vi "Periodic Tasks.vi"(8 "error in":errorcluster) -> ()   [LabVIEW 2020]
doc: "This VI runs in parallel to other tasks. It can contain as many user-defined periodic loops as you need. These can carry out PID or other sorts of timed response."
uses:
  <vilib>/Rock Robotics/WPI/Utilities/WPI_GetSetVariantRefNum.vi
  Global Shooter Speed.vi
  <vilib>/Rock Robotics/WPI/ThirdParty/Phoenix-LabVIEW/CANCoder/Get/CTRE_Phoenix_CANcoder_GetSensorData.vi
  Auto Variables.vi
  <vilib>/Rock Robotics/Network Tables/NT Write Number.vi
panel:
  out "Gyro Angle":dbl
  # "Click here to set min"
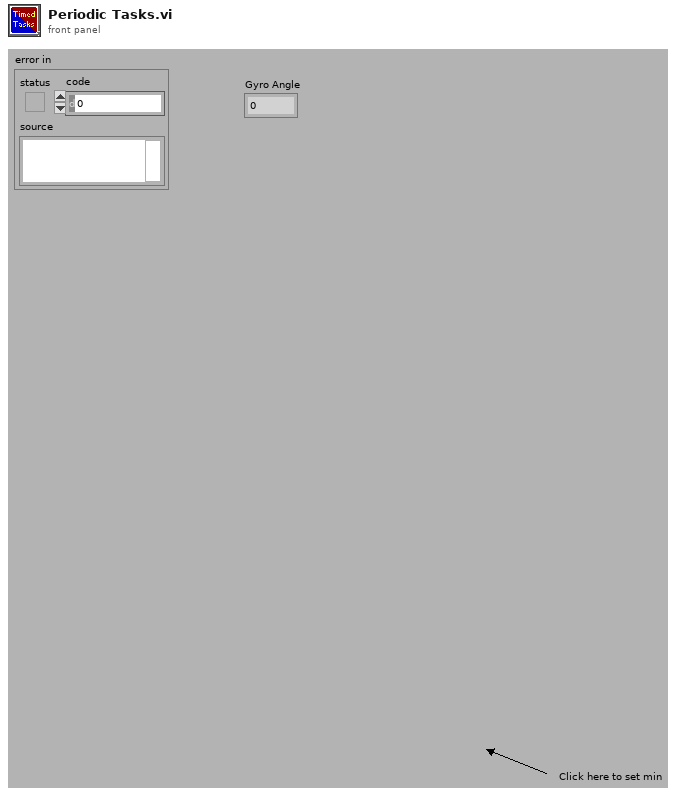
[diagram p1: front panel]
types:
  T1 = typedef "WPI_JoystickDevRef.ctl" = cluster{"Device":T2}
  T2 = typedef "WPI_JoystickDeviceEnum.ctl" = enum16{"USB 0", "USB 1", "USB 2", "USB 3", "USB 4", "USB 5"}
  T3 = typedef "WPI_RobotDriveDevRef.ctl" = cluster{"DevStatus":errorcluster, "Motors[]":T4[], "Square Inputs":bool, "Max Output":dbl}
  T4 = typedef "WPI_MotorControlDeviceRef.ctl" = cluster{"DeviceStatus":errorcluster, "Type":T5, "PWM":cluster{"PWM Channel":T6, "DeadBand":T7}, "CAN":cluster{"Device Number":u8, "SetOutput VI Ref":variant, "GetOutput VI Ref":variant, "Enable VI Ref":variant, "Disable VI Ref":variant, "Data":variant}, "Invert":bool, "DIO PWM":cluster{"PWM \"Enable\" Channel":T6, "DIOChannel":T8, "PWM Rate":dbl}}
  T5 = typedef "WPI_MotorControlType.ctl" = enum16{"PWM", "CAN", "DIO PWM"}
  T6 = typedef "FPGA_DIOPWMChannel.ctl" = enum8{"PWM 0", "PWM 1", "PWM 2", "PWM 3", "PWM 4", "PWM 5", "PWM 6", "PWM 7", "PWM 8", "PWM 9", "PWM MXP 0", "PWM MXP 1", "PWM MXP 2", "PWM MXP 3", "PWM MXP 4", "PWM MXP 5", "PWM MXP 6", "PWM MXP 7", "PWM MXP 8", "PWM MXP 9", "Invalid"}
  T7 = typedef "WPI_PWMDeadband.ctl" = cluster{"Name":string, "maxPositivePwm":i32, "minPositivePwm":i32, "centerPwm":i32, "maxNegativePwm":i32, "minNegativePwm":i32, "angularRange":u16}
  T8 = typedef "FPGA_DIOChannel.ctl" = enum8{"DIO 0", "DIO 1", "DIO 2", "DIO 3", "DIO 4", "DIO 5", "DIO 6", "DIO 7", "DIO 8", "DIO 9", "DIO MXP 0", "DIO MXP 1", "DIO MXP 2", "DIO MXP 3", "DIO MXP 4", "DIO MXP 5", "DIO MXP 6", "DIO MXP 7", "DIO MXP 8", "DIO MXP 9", "DIO MXP 10", "DIO MXP 11", "DIO MXP 12", "DIO MXP 13", "DIO MXP 14", "DIO MXP 15", "SPI Port CS1", "SPI Port CS2", "SPI Port CS3", "SPI Port MISO", "SPI Port MOSI", "Invalid"}
  T9 = typedef "CTRE_Phoenix_CANcoder_DeviceRef.ctl" = cluster{"DeviceStatus":errorcluster, "Device Number":u8, "Handle":u64, "UsageFrame":u32, "Library Path":path}
  T10 = cluster{"MotorControlDevRef":T4, "MotorControlDevRef":T4, "MotorControlDevRef":T4}
  T11 = cluster{"JoystickDevRef":T1, "JoystickDevRef":T1, "RobotDriveDevRef":T3}
  T12 = typedef "WPI_GyroDevRef.ctl" = cluster{"DevStatus":errorcluster, "Analog Channel":T13, "Gain (VoltsPerDegree/Second)":dbl, "Gyro Type":enum16{"Analog", "XRS450"}, "Handle":i32, "SPI Bus":T14, "Device Found":bool, "Sample Rate":dbl, "Calibrate On Open":bool, "Offset":dbl}
  T13 = typedef "FPGA_AIChannel.ctl" = enum8{"AI 0", "AI 1", "AI 2", "AI 3", "AI MXP 0", "AI MXP 1", "AI MXP 2", "AI MXP 3", "Invalid"}
  T14 = typedef "spi_bus.ctl" = enum16{"SPI On-Board, CS0", "SPI On-Board, CS1", "SPI On-Board, CS2", "SPI On-Board, CS3", "SPI MXP", "Invalid"}
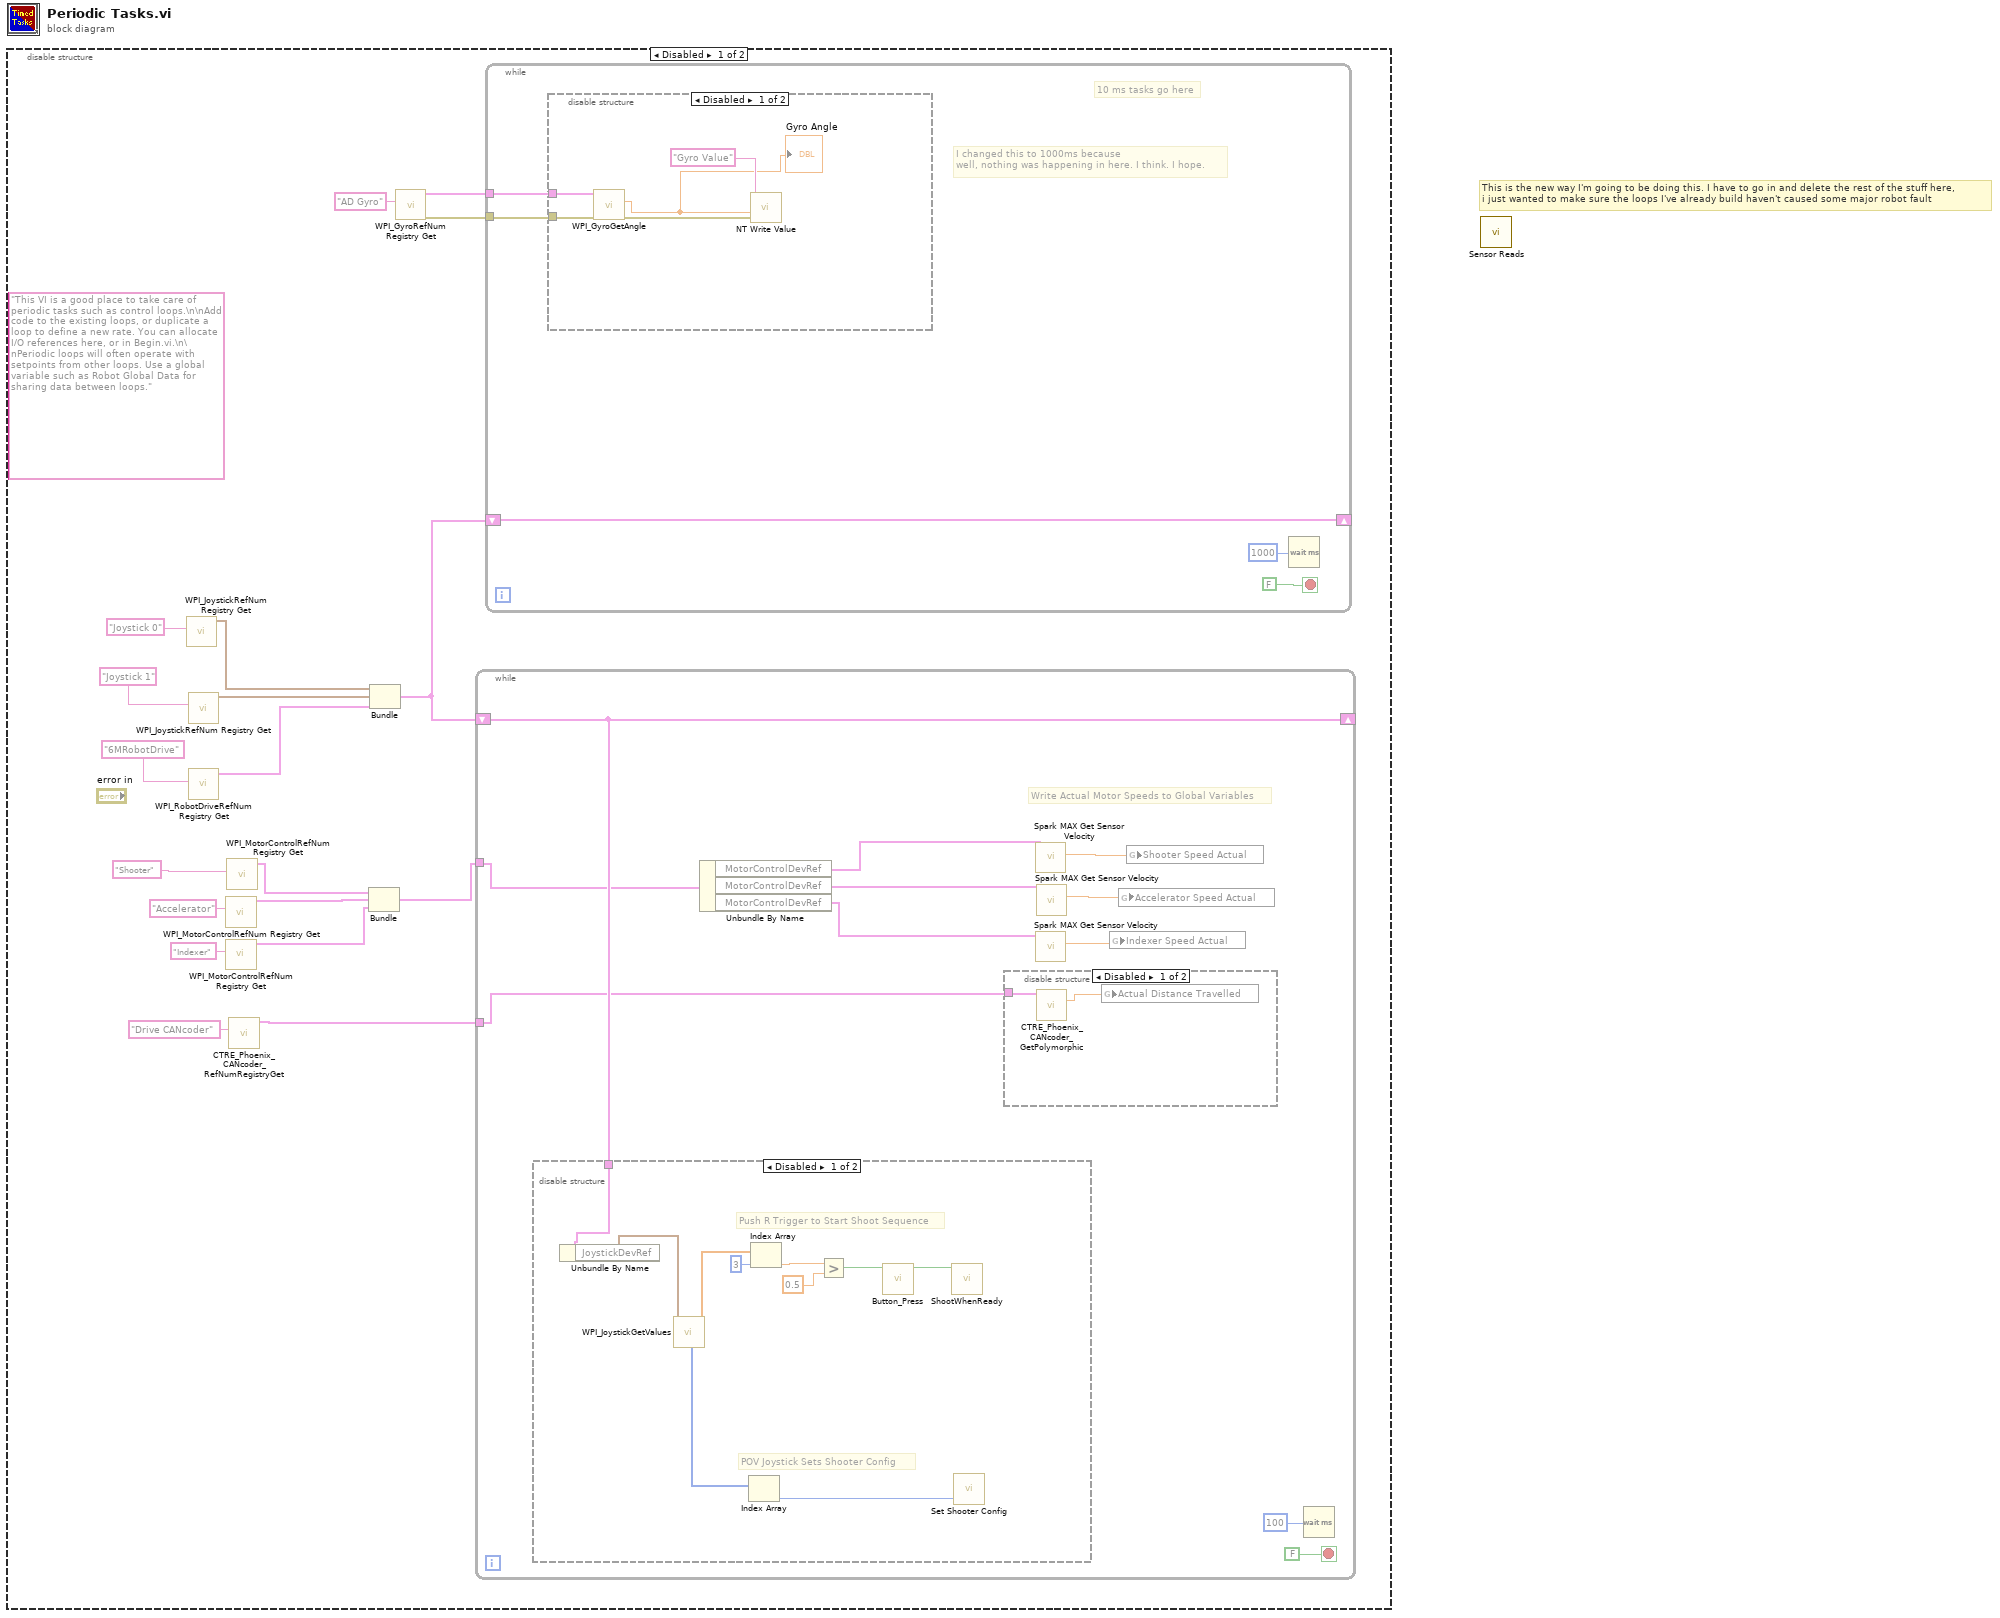
[diagram p0: block diagram]
diagram:
  # "This is the new way I'm going to be doing this. I have to go in and delete the rest of the stuff here,\ni just wanted to make sure the loops I've already build haven't caused some major robot fault"
  n1 = disable-structure shown="Disabled" {
    frame Disabled {
      (unwired) "This VI is a good place to take care of periodic tasks such as control loops.\n\nAdd code to the existing loops, or duplicate a loop to define a new rate. You can allocate I/O references here, or in Begin.vi.\n\nPeriodic loops will often operate with setpoints from other loops. Use a global variable such as Robot Global Data for sharing data between loops."
      n2 = call <vilib>:"WPI_JoystickRefNum Registry Get.vi"("refnum name"="Joystick 0") -> ("JoystickDevRef"=w13:T1)  [unwired: 9 in, 1 out]
      n3 = call <vilib>:"WPI_JoystickRefNum Registry Get.vi"("refnum name"="Joystick 1") -> ("JoystickDevRef"=w17:T1)  [unwired: 1 in, 9 out]
      n4 = call <vilib>:"WPI_RobotDriveRefNum Registry Get.vi"("refnum name"="6MRobotDrive") -> ("RobotDriveDevRef"=w16:T3)  [unwired: 1 in, 9 out]
      n5 = call <vilib>:"WPI_MotorControlRefNum Registry Get.vi"("refnum name"="Accelerator") -> ("MotorControlDevRef"=w6:T4)  [unwired: 9 in, 1 out]
      n6 = call <vilib>:"WPI_MotorControlRefNum Registry Get.vi"("refnum name"="Indexer") -> ("MotorControlDevRef"=w5:T4)  [unwired: 9 in, 1 out]
      n7 = call <vilib>:"WPI_MotorControlRefNum Registry Get.vi"("refnum name"="Shooter") -> ("MotorControlDevRef"=w7:T4)  [unwired: 9 in, 1 out]
      n8 = call <vilib>:"CTRE_Phoenix_CANcoder_RefNumRegistryGet.vi"("refnum name"="Drive CANcoder") -> ("CTRE_CANcoder_DeviceRef"=w8:T9)  [unwired: 9 in, 1 out]
      n9 = Bundle("MotorControlDevRef"=w7, "MotorControlDevRef"=w6, "MotorControlDevRef"=w5) -> (w4:T10)  [unwired: 1 in]
      n10 = Bundle("JoystickDevRef"=w13, "JoystickDevRef"=w17, "RobotDriveDevRef"=w16) -> (w15:T11)  [unwired: 1 out]
      n11 = call <vilib>:"WPI_GyroRefNum Registry Get.vi"("refnum name"="AD Gyro") -> ("error out"=w1:errorcluster, "GyroDevRef"=w2:T12)  [unwired: 9 in]
      n12 = while {
        shift-right: [w28] -> _
        shift-left: w15 -> [w28]
        tunnel: w4 -> [w23]
        tunnel: w8 -> [w24]
        stop <- FALSE stop-if-true
        # "Write Actual Motor Speeds to Global Variables"
        n13 = disable-structure shown="Disabled" {
          disable-tunnel: w28 -> [w40 _]
          frame Disabled {
            # "Push R Trigger to Start Shoot Sequence"
            # "POV Joystick Sets Shooter Config"
            n14 = Unbundle By Name(w40) -> ("JoystickDevRef"=w39:T1)
            n15 = call <vilib>:"WPI_JoystickGetValues.vi"("JoystickDevRef"=w39) -> ("Axes"=w36:dbl[], "POVs"=w38:i16[])  [unwired: 6 in, 3 out]
            n16 = Index Array(array=w38) -> (element=w37:i16)  [unwired: 1 in]
            n17 = Index Array(array=w36, index=3) -> (element=w34:dbl)
            n18 = Greater?(x=w34, y=0.5) -> (0:w32:bool)
            n19 = call "Button_Press.vi"("Button In"=w32) -> ("Button Pressed?"=w31:bool)  [unwired: 10 in]
            n20 = call "ShootWhenReady.vi"("Start Shooting"=w31) -> ()  [unwired: 11 in]
            n21 = call "Set Shooter Config.vi"("POV Joystick Input"=w37) -> ()  [unwired: 3 in]
          }
          frame Enabled {
          }
        }
        n22 = Unbundle By Name(w23) -> ("MotorControlDevRef"=w22:T4, "MotorControlDevRef"=w21:T4, "MotorControlDevRef"=w20:T4)
        n23 = disable-structure shown="Disabled" {
          disable-tunnel: w24 -> [w42 _]
          frame Disabled {
            n24 = call-poly <vilib>:"CTRE_Phoenix_CANcoder_GetPolymorphic.vi"("CTRE_CANcoder_DeviceRef"=w42) -> ("Position"=w41:dbl)  [unwired: 10 in, 4 out]
            n25 = global write "Auto Variables.vi" "Actual Distance Travelled"(w41) -> ()
          }
          frame Enabled {
          }
        }
        n26 = call <vilib>:"Spark MAX Get Sensor Velocity.vi"("MotorControlDevRef in"=w22) -> ("Sensor Velocity"=w27:dbl)  [unwired: 7 in, 3 out]
        n27 = call <vilib>:"Spark MAX Get Sensor Velocity.vi"("MotorControlDevRef in"=w20) -> ("Sensor Velocity"=w25:dbl)  [unwired: 7 in, 3 out]
        n28 = call <vilib>:"Spark MAX Get Sensor Velocity.vi"("MotorControlDevRef in"=w21) -> ("Sensor Velocity"=w26:dbl)  [unwired: 7 in, 3 out]
        n29 = global write "Global Shooter Speed.vi" "Indexer Speed Actual"(w25) -> ()
        n30 = global write "Global Shooter Speed.vi" "Accelerator Speed Actual"(w26) -> ()
        n31 = global write "Global Shooter Speed.vi" "Shooter Speed Actual"(w27) -> ()
        n32 = Wait (ms)(milliseconds to wait=u32 100) -> ()  [unwired: 1 out]
      }
      n33 = while {
        shift-right: [w45] -> _
        shift-left: w15 -> [w45]
        tunnel: w2 -> [w44]
        tunnel: w1 -> [w43]
        stop <- FALSE stop-if-true
        # "I changed this to 1000ms because\nwell, nothing was happening in here. I think. I hope."
        # "10 ms tasks go here"
        n34 = disable-structure shown="Disabled" {
          disable-tunnel: w44 -> [w52 _]
          disable-tunnel: w43 -> [w51 _]
          frame Disabled {
            n35 = call <vilib>:"WPI_GyroGetAngle.vi"("error in (no error)"=w51, "GyroDevRef"=w52) -> ("error out"=w49:errorcluster, "Angle"=w48:dbl)  [unwired: 5 in, 3 out]
            "Gyro Angle" <- w48
            n36 = call-poly <vilib>:"NT Write Value.vi"("error in"=w49, "Numeric"=w48, "Name"="Gyro Value") -> ()  [unwired: 8 in, 1 out]
          }
          frame Enabled {
          }
        }
        n37 = Wait (ms)(milliseconds to wait=u32 1000) -> ()  [unwired: 1 out]
      }
    }
    frame Enabled {
    }
  }
  n38 = call "Sensor Reads.vi"() -> ()  [unwired: 12 in]
